vi "VAT_valve_shut.vi"(0 "VAT Valve COM port":refnum<visa-resource-name>, 2 "Unit":string, 11 "error in (no error)":errorcluster) -> (4 "VAT Valve COM port out":refnum<visa-resource-name>, 13 "Valve Position":dbl=0.000499, 15 "error out":errorcluster)   [LabVIEW 2019]
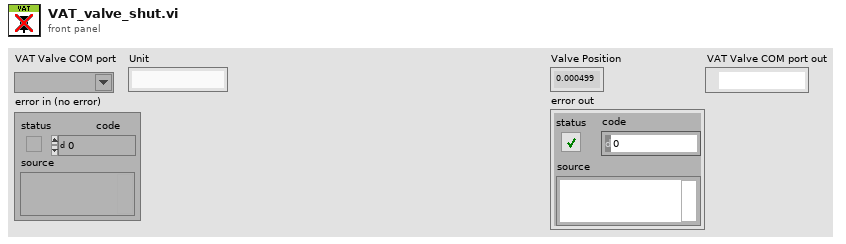
[diagram p1: front panel]
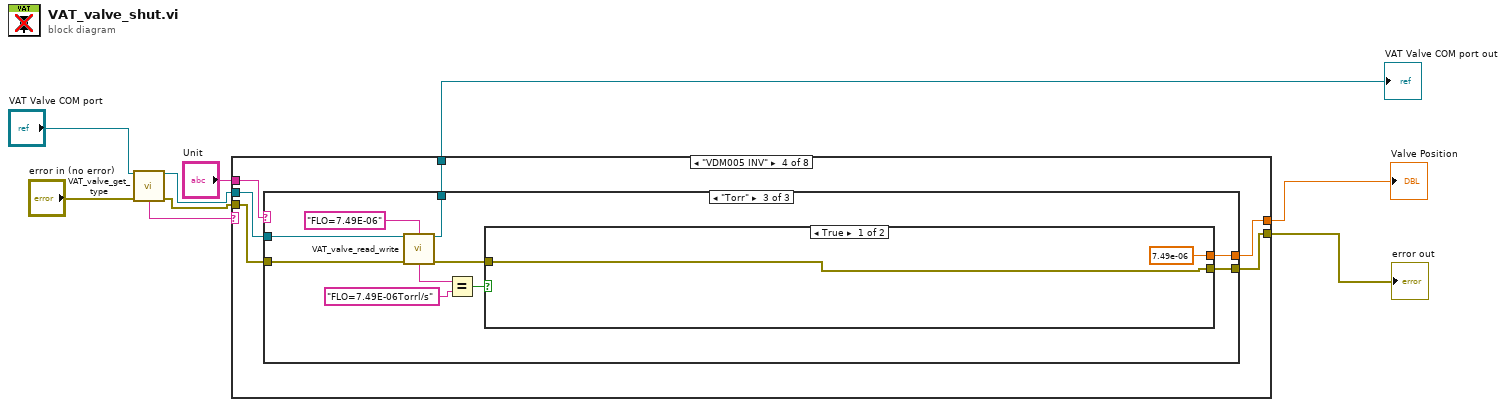
[diagram p0: block diagram]
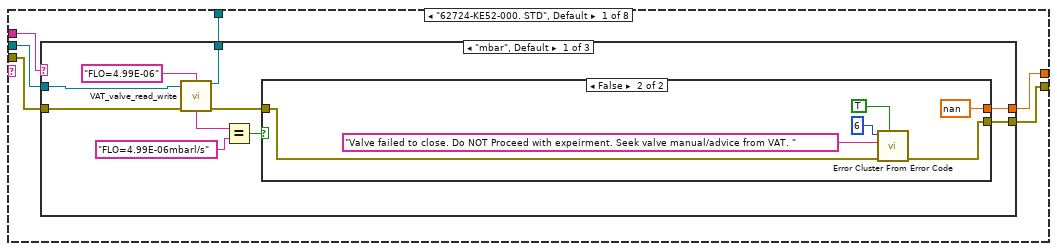
[diagram p2: hidden frame]
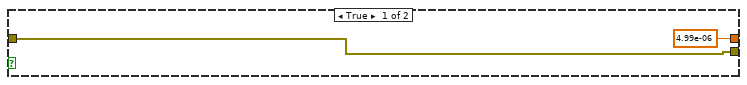
[diagram p3: hidden frame]
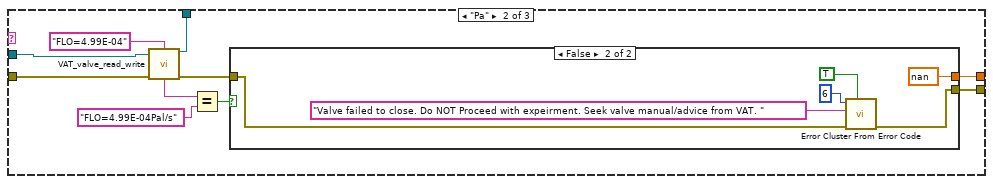
[diagram p4: hidden frame]
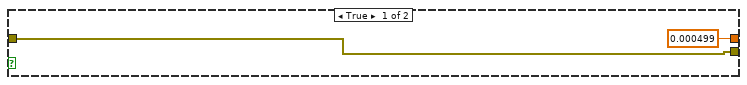
[diagram p5: hidden frame]
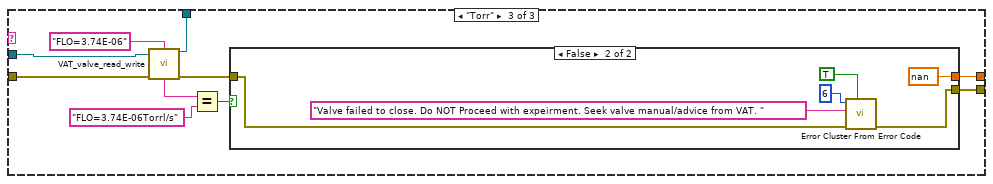
[diagram p6: hidden frame]
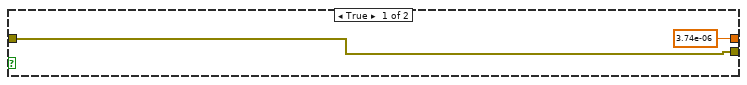
[diagram p7: hidden frame]
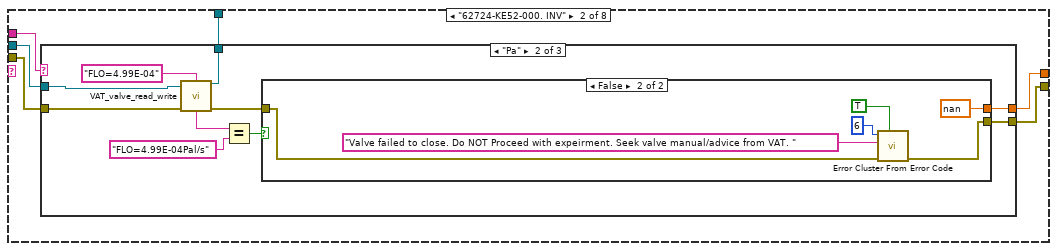
[diagram p8: hidden frame]
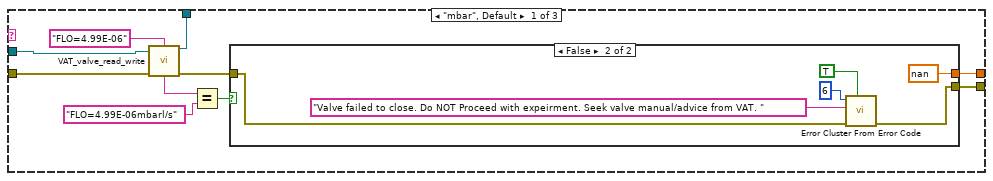
[diagram p9: hidden frame]
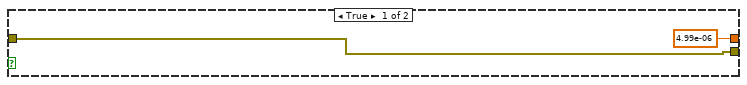
[diagram p10: hidden frame]
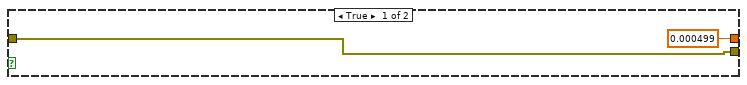
[diagram p11: hidden frame]
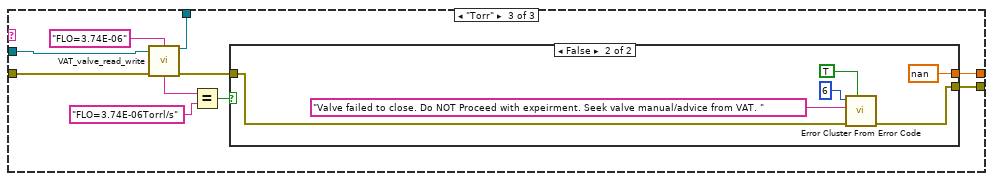
[diagram p12: hidden frame]
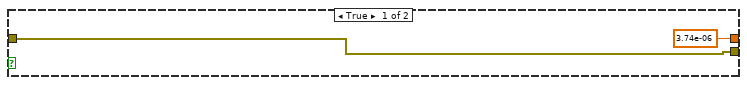
[diagram p13: hidden frame]
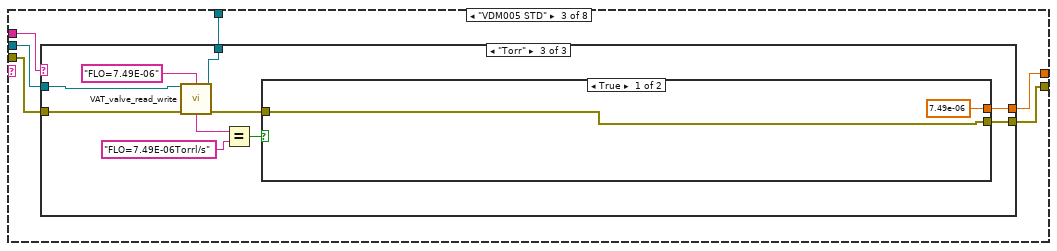
[diagram p14: hidden frame]
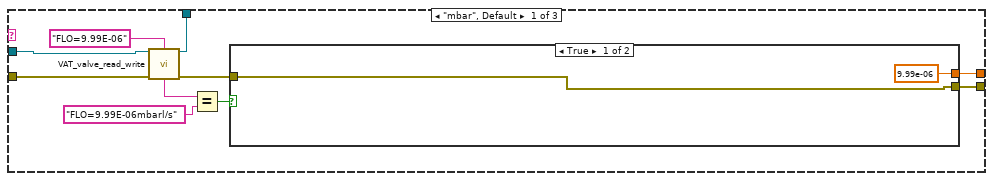
[diagram p15: hidden frame]
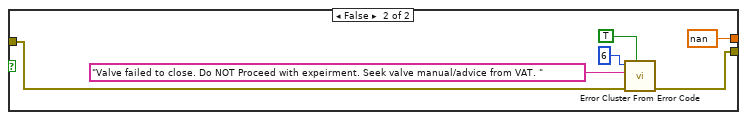
[diagram p16: hidden frame]
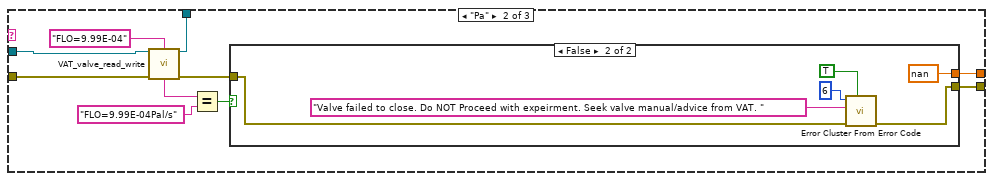
[diagram p17: hidden frame]
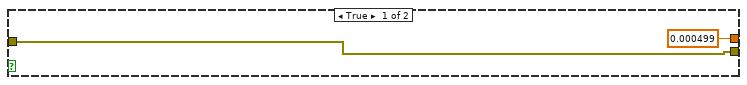
[diagram p18: hidden frame]
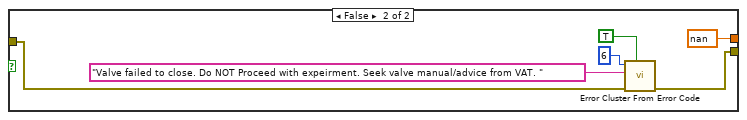
[diagram p19: hidden frame]
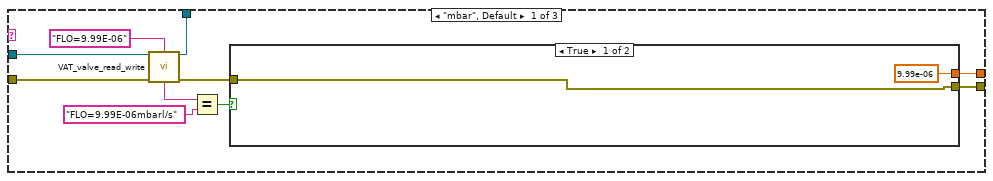
[diagram p20: hidden frame]
diagram:
  n1 = call "VAT_valve_get_type.vi"("VAT Valve COM port"="VAT Valve COM port", "error in (no error)"="error in (no error)") -> ("VAT Valve COM port out"=w6:refnum<visa-resource-name>, "Valve Type"=w5:string, "error out"=w7:errorcluster)  [unwired: 11 in]
  n2 = case shown="\"VDM005 INV\"" w5 {
    tunnel: w6 -> [w15 w75 w135 w195 w259 w277 w295 w313]
    tunnel: w7 -> [w14 w74 w134 w194 w258 w276 w294 w312]
    tunnel: "Unit" -> [w13 w73 w133 w193 _ _ _ _]
    tunnel: [w12 w72 w132 w192 w252 w270 w288 w306] -> w3
    tunnel: [w11 w71 w131 w191 w253 w271 w289 w307] -> w2
    tunnel: [w10 w70 w130 w190 w250 w268 w286 w304] -> w1
    frame "62724-KE52-000. STD", Default {
      n3 = case shown="\"mbar\", Default" w13 {
        tunnel: w15 -> [w25 w43 w61]
        tunnel: w14 -> [w24 w42 w60]
        tunnel: [w18 w36 w54] -> w12
        tunnel: [w17 w35 w53] -> w11
        tunnel: [w16 w34 w52] -> w10
        frame "mbar", Default {
          n4 = call "VAT_valve_read_write.vi"("VAT Valve COM port"=w25, "Write String"="FLO=4.99E-06", "error in (no error)"=w24) -> ("VAT Valve COM port out"=w16:refnum<visa-resource-name>, "Read String"=w21:string, "error out"=w19:errorcluster)  [unwired: 10 in]
          n5 = Equal?(x=w21, y="FLO=4.99E-06mbarl/s") -> (x = y?=w22:bool)
          n6 = case shown="False" w22 {
            tunnel: w19 -> [w27 w33]
            tunnel: [w27 w29] -> w17
            tunnel: [4.99e-06 nan] -> w18
            frame True {
            }
            frame False {
              n7 = call <vilib>:"Error Cluster From Error Code.vi"("show call chain? (False)"=TRUE, "error in (no error)"=w33, "error message (\"\")"="Valve failed to close. Do NOT Proceed with expeirment. Seek valve manual/advice from VAT. " ("error message (\"\")"), "error code (0)"=6) -> ("error out"=w29:errorcluster)  [unwired: 5 in]
            }
          }
        }
        frame "Pa" {
          n8 = call "VAT_valve_read_write.vi"("VAT Valve COM port"=w43, "Write String"="FLO=4.99E-04", "error in (no error)"=w42) -> ("VAT Valve COM port out"=w34:refnum<visa-resource-name>, "Read String"=w39:string, "error out"=w37:errorcluster)  [unwired: 10 in]
          n9 = Equal?(x=w39, y="FLO=4.99E-04Pal/s") -> (x = y?=w40:bool)
          n10 = case shown="False" w40 {
            tunnel: w37 -> [w45 w51]
            tunnel: [w45 w47] -> w35
            tunnel: [0.000499 nan] -> w36
            frame True {
            }
            frame False {
              n11 = call <vilib>:"Error Cluster From Error Code.vi"("show call chain? (False)"=TRUE, "error in (no error)"=w51, "error message (\"\")"="Valve failed to close. Do NOT Proceed with expeirment. Seek valve manual/advice from VAT. " ("error message (\"\")"), "error code (0)"=6) -> ("error out"=w47:errorcluster)  [unwired: 5 in]
            }
          }
        }
        frame "Torr" {
          n12 = call "VAT_valve_read_write.vi"("VAT Valve COM port"=w61, "Write String"="FLO=3.74E-06", "error in (no error)"=w60) -> ("VAT Valve COM port out"=w52:refnum<visa-resource-name>, "Read String"=w57:string, "error out"=w55:errorcluster)  [unwired: 10 in]
          n13 = Equal?(x=w57, y="FLO=3.74E-06Torrl/s") -> (x = y?=w58:bool)
          n14 = case shown="False" w58 {
            tunnel: w55 -> [w63 w69]
            tunnel: [w63 w65] -> w53
            tunnel: [3.74e-06 nan] -> w54
            frame True {
            }
            frame False {
              n15 = call <vilib>:"Error Cluster From Error Code.vi"("show call chain? (False)"=TRUE, "error in (no error)"=w69, "error message (\"\")"="Valve failed to close. Do NOT Proceed with expeirment. Seek valve manual/advice from VAT. " ("error message (\"\")"), "error code (0)"=6) -> ("error out"=w65:errorcluster)  [unwired: 5 in]
            }
          }
        }
      }
    }
    frame "62724-KE52-000. INV" {
      n16 = case shown="\"Pa\"" w73 {
        tunnel: w75 -> [w85 w103 w121]
        tunnel: w74 -> [w84 w102 w120]
        tunnel: [w78 w96 w114] -> w72
        tunnel: [w77 w95 w113] -> w71
        tunnel: [w76 w94 w112] -> w70
        frame "mbar", Default {
          n17 = call "VAT_valve_read_write.vi"("VAT Valve COM port"=w85, "Write String"="FLO=4.99E-06", "error in (no error)"=w84) -> ("VAT Valve COM port out"=w76:refnum<visa-resource-name>, "Read String"=w81:string, "error out"=w79:errorcluster)  [unwired: 10 in]
          n18 = Equal?(x=w81, y="FLO=4.99E-06mbarl/s") -> (x = y?=w82:bool)
          n19 = case shown="False" w82 {
            tunnel: w79 -> [w87 w93]
            tunnel: [w87 w89] -> w77
            tunnel: [4.99e-06 nan] -> w78
            frame True {
            }
            frame False {
              n20 = call <vilib>:"Error Cluster From Error Code.vi"("show call chain? (False)"=TRUE, "error in (no error)"=w93, "error message (\"\")"="Valve failed to close. Do NOT Proceed with expeirment. Seek valve manual/advice from VAT. " ("error message (\"\")"), "error code (0)"=6) -> ("error out"=w89:errorcluster)  [unwired: 5 in]
            }
          }
        }
        frame "Pa" {
          n21 = call "VAT_valve_read_write.vi"("VAT Valve COM port"=w103, "Write String"="FLO=4.99E-04", "error in (no error)"=w102) -> ("VAT Valve COM port out"=w94:refnum<visa-resource-name>, "Read String"=w99:string, "error out"=w97:errorcluster)  [unwired: 10 in]
          n22 = Equal?(x=w99, y="FLO=4.99E-04Pal/s") -> (x = y?=w100:bool)
          n23 = case shown="False" w100 {
            tunnel: w97 -> [w105 w111]
            tunnel: [w105 w107] -> w95
            tunnel: [0.000499 nan] -> w96
            frame True {
            }
            frame False {
              n24 = call <vilib>:"Error Cluster From Error Code.vi"("show call chain? (False)"=TRUE, "error in (no error)"=w111, "error message (\"\")"="Valve failed to close. Do NOT Proceed with expeirment. Seek valve manual/advice from VAT. " ("error message (\"\")"), "error code (0)"=6) -> ("error out"=w107:errorcluster)  [unwired: 5 in]
            }
          }
        }
        frame "Torr" {
          n25 = call "VAT_valve_read_write.vi"("VAT Valve COM port"=w121, "Write String"="FLO=3.74E-06", "error in (no error)"=w120) -> ("VAT Valve COM port out"=w112:refnum<visa-resource-name>, "Read String"=w117:string, "error out"=w115:errorcluster)  [unwired: 10 in]
          n26 = Equal?(x=w117, y="FLO=3.74E-06Torrl/s") -> (x = y?=w118:bool)
          n27 = case shown="False" w118 {
            tunnel: w115 -> [w123 w129]
            tunnel: [w123 w125] -> w113
            tunnel: [3.74e-06 nan] -> w114
            frame True {
            }
            frame False {
              n28 = call <vilib>:"Error Cluster From Error Code.vi"("show call chain? (False)"=TRUE, "error in (no error)"=w129, "error message (\"\")"="Valve failed to close. Do NOT Proceed with expeirment. Seek valve manual/advice from VAT. " ("error message (\"\")"), "error code (0)"=6) -> ("error out"=w125:errorcluster)  [unwired: 5 in]
            }
          }
        }
      }
    }
    frame "VDM005 STD" {
      n29 = case shown="\"Torr\"" w133 {
        tunnel: w135 -> [w145 w163 w181]
        tunnel: w134 -> [w144 w162 w180]
        tunnel: [w138 w156 w174] -> w132
        tunnel: [w137 w155 w173] -> w131
        tunnel: [w136 w154 w172] -> w130
        frame "mbar", Default {
          n30 = call "VAT_valve_read_write.vi"("VAT Valve COM port"=w145, "Write String"="FLO=9.99E-06", "error in (no error)"=w144) -> ("VAT Valve COM port out"=w136:refnum<visa-resource-name>, "Read String"=w141:string, "error out"=w139:errorcluster)  [unwired: 10 in]
          n31 = Equal?(x=w141, y="FLO=9.99E-06mbarl/s") -> (x = y?=w142:bool)
          n32 = case shown="True" w142 {
            tunnel: w139 -> [w147 w153]
            tunnel: [w147 w149] -> w137
            tunnel: [9.99e-06 nan] -> w138
            frame True {
            }
            frame False {
              n33 = call <vilib>:"Error Cluster From Error Code.vi"("show call chain? (False)"=TRUE, "error in (no error)"=w153, "error message (\"\")"="Valve failed to close. Do NOT Proceed with expeirment. Seek valve manual/advice from VAT. " ("error message (\"\")"), "error code (0)"=6) -> ("error out"=w149:errorcluster)  [unwired: 5 in]
            }
          }
        }
        frame "Pa" {
          n34 = call "VAT_valve_read_write.vi"("VAT Valve COM port"=w163, "Write String"="FLO=9.99E-04", "error in (no error)"=w162) -> ("VAT Valve COM port out"=w154:refnum<visa-resource-name>, "Read String"=w159:string, "error out"=w157:errorcluster)  [unwired: 10 in]
          n35 = Equal?(x=w159, y="FLO=9.99E-04Pal/s") -> (x = y?=w160:bool)
          n36 = case shown="False" w160 {
            tunnel: w157 -> [w165 w171]
            tunnel: [w165 w167] -> w155
            tunnel: [0.000499 nan] -> w156
            frame True {
            }
            frame False {
              n37 = call <vilib>:"Error Cluster From Error Code.vi"("show call chain? (False)"=TRUE, "error in (no error)"=w171, "error message (\"\")"="Valve failed to close. Do NOT Proceed with expeirment. Seek valve manual/advice from VAT. " ("error message (\"\")"), "error code (0)"=6) -> ("error out"=w167:errorcluster)  [unwired: 5 in]
            }
          }
        }
        frame "Torr" {
          n38 = call "VAT_valve_read_write.vi"("VAT Valve COM port"=w181, "Write String"="FLO=7.49E-06", "error in (no error)"=w180) -> ("VAT Valve COM port out"=w172:refnum<visa-resource-name>, "Read String"=w177:string, "error out"=w175:errorcluster)  [unwired: 10 in]
          n39 = Equal?(x=w177, y="FLO=7.49E-06Torrl/s") -> (x = y?=w178:bool)
          n40 = case shown="True" w178 {
            tunnel: w175 -> [w183 w189]
            tunnel: [w183 w185] -> w173
            tunnel: [7.49e-06 nan] -> w174
            frame True {
            }
            frame False {
              n41 = call <vilib>:"Error Cluster From Error Code.vi"("show call chain? (False)"=TRUE, "error in (no error)"=w189, "error message (\"\")"="Valve failed to close. Do NOT Proceed with expeirment. Seek valve manual/advice from VAT. " ("error message (\"\")"), "error code (0)"=6) -> ("error out"=w185:errorcluster)  [unwired: 5 in]
            }
          }
        }
      }
    }
    frame "VDM005 INV" {
      n42 = case shown="\"Torr\"" w193 {
        tunnel: w195 -> [w205 w223 w241]
        tunnel: w194 -> [w204 w222 w240]
        tunnel: [w198 w216 w234] -> w192
        tunnel: [w197 w215 w233] -> w191
        tunnel: [w196 w214 w232] -> w190
        frame "mbar", Default {
          n43 = call "VAT_valve_read_write.vi"("VAT Valve COM port"=w205, "Write String"="FLO=9.99E-06", "error in (no error)"=w204) -> ("VAT Valve COM port out"=w196:refnum<visa-resource-name>, "Read String"=w201:string, "error out"=w199:errorcluster)  [unwired: 10 in]
          n44 = Equal?(x=w201, y="FLO=9.99E-06mbarl/s") -> (x = y?=w202:bool)
          n45 = case shown="True" w202 {
            tunnel: w199 -> [w207 w213]
            tunnel: [w207 w209] -> w197
            tunnel: [9.99e-06 nan] -> w198
            frame True {
            }
            frame False {
              n46 = call <vilib>:"Error Cluster From Error Code.vi"("show call chain? (False)"=TRUE, "error in (no error)"=w213, "error message (\"\")"="Valve failed to close. Do NOT Proceed with expeirment. Seek valve manual/advice from VAT. " ("error message (\"\")"), "error code (0)"=6) -> ("error out"=w209:errorcluster)  [unwired: 5 in]
            }
          }
        }
        frame "Pa" {
          n47 = call "VAT_valve_read_write.vi"("VAT Valve COM port"=w223, "Write String"="FLO=9.99E-04", "error in (no error)"=w222) -> ("VAT Valve COM port out"=w214:refnum<visa-resource-name>, "Read String"=w219:string, "error out"=w217:errorcluster)  [unwired: 10 in]
          n48 = Equal?(x=w219, y="FLO=9.99E-04Pal/s") -> (x = y?=w220:bool)
          n49 = case shown="False" w220 {
            tunnel: w217 -> [w225 w231]
            tunnel: [w225 w227] -> w215
            tunnel: [0.000499 nan] -> w216
            frame True {
            }
            frame False {
              n50 = call <vilib>:"Error Cluster From Error Code.vi"("show call chain? (False)"=TRUE, "error in (no error)"=w231, "error message (\"\")"="Valve failed to close. Do NOT Proceed with expeirment. Seek valve manual/advice from VAT. " ("error message (\"\")"), "error code (0)"=6) -> ("error out"=w227:errorcluster)  [unwired: 5 in]
            }
          }
        }
        frame "Torr" {
          n51 = call "VAT_valve_read_write.vi"("VAT Valve COM port"=w241, "Write String"="FLO=7.49E-06", "error in (no error)"=w240) -> ("VAT Valve COM port out"=w232:refnum<visa-resource-name>, "Read String"=w237:string, "error out"=w235:errorcluster)  [unwired: 10 in]
          n52 = Equal?(x=w237, y="FLO=7.49E-06Torrl/s") -> (x = y?=w238:bool)
          n53 = case shown="True" w238 {
            tunnel: w235 -> [w243 w249]
            tunnel: [w243 w245] -> w233
            tunnel: [7.49e-06 nan] -> w234
            frame True {
            }
            frame False {
              n54 = call <vilib>:"Error Cluster From Error Code.vi"("show call chain? (False)"=TRUE, "error in (no error)"=w249, "error message (\"\")"="Valve failed to close. Do NOT Proceed with expeirment. Seek valve manual/advice from VAT. " ("error message (\"\")"), "error code (0)"=6) -> ("error out"=w245:errorcluster)  [unwired: 5 in]
            }
          }
        }
      }
    }
    frame "AA 2 STD" {
      n55 = call "VAT_valve_read_write.vi"("VAT Valve COM port"=w259, "Write String"="FLO=00000", "error in (no error)"=w258) -> ("VAT Valve COM port out"=w250:refnum<visa-resource-name>, "Read String"=w256:string, "error out"=w251:errorcluster)  [unwired: 10 in]
      n56 = Equal?(x=w256, y="FLO=\\s\\s\\s\\s0mV%") -> (x = y?=w254:bool)
      n57 = case shown="False" w254 {
        tunnel: [w261 w265] -> w253
        tunnel: [0.0 nan] -> w252
        tunnel: w251 -> [w261 w263]
        frame True {
        }
        frame False {
          n58 = call <vilib>:"Error Cluster From Error Code.vi"("show call chain? (False)"=TRUE, "error in (no error)"=w263, "error message (\"\")"="Valve failed to close. Do NOT Proceed with expeirment. Seek valve manual/advice from VAT. " ("error message (\"\")"), "error code (0)"=6) -> ("error out"=w265:errorcluster)  [unwired: 5 in]
        }
      }
    }
    frame "AA 2 INV" {
      n59 = call "VAT_valve_read_write.vi"("VAT Valve COM port"=w277, "Write String"="FLO=00000", "error in (no error)"=w276) -> ("VAT Valve COM port out"=w268:refnum<visa-resource-name>, "Read String"=w274:string, "error out"=w269:errorcluster)  [unwired: 10 in]
      n60 = Equal?(x=w274, y="FLO=\\s\\s\\s\\s0mV%") -> (x = y?=w272:bool)
      n61 = case shown="False" w272 {
        tunnel: [w279 w283] -> w271
        tunnel: [0.0 nan] -> w270
        tunnel: w269 -> [w279 w281]
        frame True {
        }
        frame False {
          n62 = call <vilib>:"Error Cluster From Error Code.vi"("show call chain? (False)"=TRUE, "error in (no error)"=w281, "error message (\"\")"="Valve failed to close. Do NOT Proceed with expeirment. Seek valve manual/advice from VAT. " ("error message (\"\")"), "error code (0)"=6) -> ("error out"=w283:errorcluster)  [unwired: 5 in]
        }
      }
    }
    frame "62714-.E64-AB STD" {
      n63 = call "VAT_valve_read_write.vi"("VAT Valve COM port"=w295, "Write String"="FLO=000.0", "error in (no error)"=w294) -> ("VAT Valve COM port out"=w286:refnum<visa-resource-name>, "Read String"=w292:string, "error out"=w287:errorcluster)  [unwired: 10 in]
      n64 = Equal?(x=w292, y="FLO=\\s\\s0.0%") -> (x = y?=w290:bool)
      n65 = case shown="True" w290 {
        tunnel: [w297 w301] -> w289
        tunnel: [0.0 nan] -> w288
        tunnel: w287 -> [w297 w299]
        frame True {
        }
        frame False {
          n66 = call <vilib>:"Error Cluster From Error Code.vi"("show call chain? (False)"=TRUE, "error in (no error)"=w299, "error message (\"\")"="Valve failed to close. Do NOT Proceed with expeirment. Seek valve manual/advice from VAT. " ("error message (\"\")"), "error code (0)"=6) -> ("error out"=w301:errorcluster)  [unwired: 5 in]
        }
      }
    }
    frame "62714-.E64-AB INV" {
      n67 = call "VAT_valve_read_write.vi"("VAT Valve COM port"=w313, "Write String"="FLO=000.0", "error in (no error)"=w312) -> ("VAT Valve COM port out"=w304:refnum<visa-resource-name>, "Read String"=w310:string, "error out"=w305:errorcluster)  [unwired: 10 in]
      n68 = Equal?(x=w310, y="FLO=\\s\\s0.0%") -> (x = y?=w308:bool)
      n69 = case shown="True" w308 {
        tunnel: [w315 w319] -> w307
        tunnel: [0.0 nan] -> w306
        tunnel: w305 -> [w315 w317]
        frame True {
        }
        frame False {
          n70 = call <vilib>:"Error Cluster From Error Code.vi"("show call chain? (False)"=TRUE, "error in (no error)"=w317, "error message (\"\")"="Valve failed to close. Do NOT Proceed with expeirment. Seek valve manual/advice from VAT. " ("error message (\"\")"), "error code (0)"=6) -> ("error out"=w319:errorcluster)  [unwired: 5 in]
        }
      }
    }
  }
  "Valve Position" <- w3
  "error out" <- w2
  "VAT Valve COM port out" <- w1
